vi "VI2 in Library.vi"(8 "search string/char (-)":string=".", 9 "string":string="This is a test string. Whatever is after full stop must be in output, separated by ','") -> (0 "String":string)   [LabVIEW 2023, in "Library.lvlib"]
uses:
  Library.lvlib
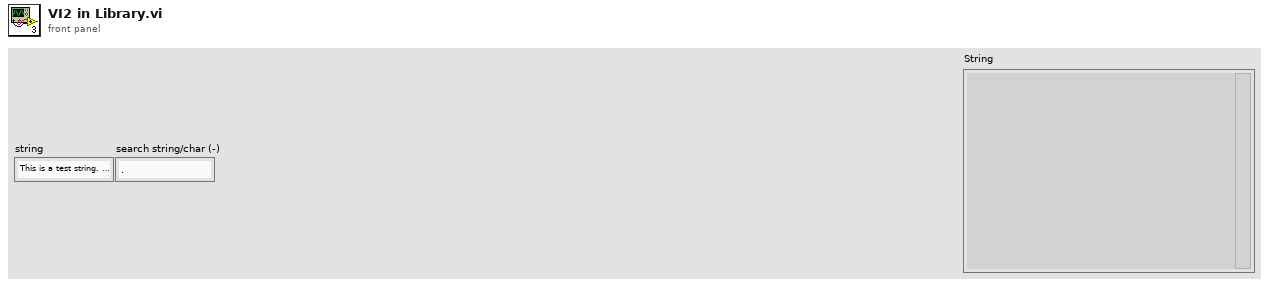
[diagram p1: front panel]
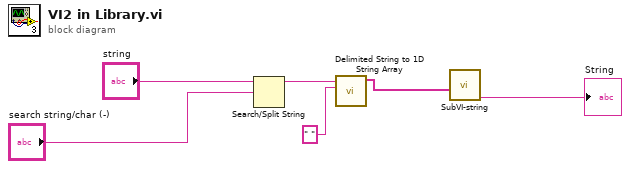
[diagram p0: block diagram]
diagram:
  n1 = Search/Split String(string="string", search string/char (-)="search string/char (-)") -> (substring before match=w4:string)  [unwired: 1 in, 2 out]
  n2 = call <vilib>:"Delimited String to 1D String Array.vi"("delimiter"=" ", "delimited string"=w4) -> ("string array"=w2:string[])  [unwired: 9 in]
  n3 = call "SubVI-string.vi"("Strings In"=w2) -> ("String"=→"String":string)  [unwired: 10 in]
